vi "RM.searchClientInfoArrayByGUID.vi"(8 "error in (no error)":errorcluster, 10 "ClientGUID":string, 11 "Client Array in":T1[](array[typedef]) {"CD Ref" format="%.0x"}) -> (0 "error out":errorcluster, 1 "found?":bool, 2 "ClientInfo":T1 {"CD Ref" format="%.0x"}, 3 "Client Array out":T1[](array[typedef]) {"CD Ref" format="%.0x"})   [LabVIEW 2016, in "FPGA Resource Manager.lvlib"]
uses:
  FPGA Resource Manager.lvlib
  RM.clientInfo.ctl
  <vilib>/NI Veristand/Custom Device API/Custom Device Item Ref.ctl
  <vilib>/NI Veristand/Custom Device API/Custom Device API.lvlib
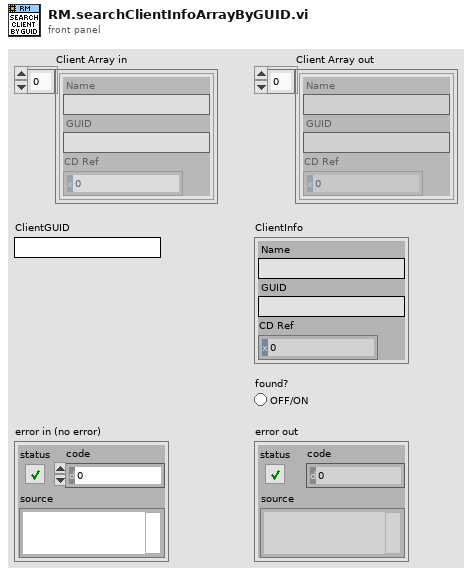
[diagram p1: front panel]
types:
  T1 = typedef "FPGA Resource Manager.lvlib/RM.clientInfo.ctl" = cluster{"Name":string, "GUID":string, "CD Ref":T2}
  T2 = typedef "Custom Device API.lvlib/Custom Device Item Ref.ctl" = u64
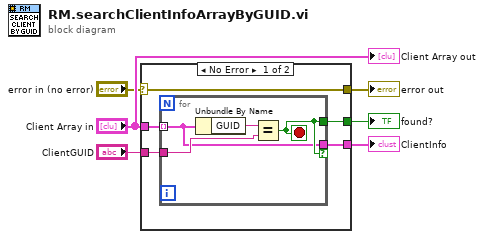
[diagram p0: block diagram]
diagram:
  n1 = case shown="No Error" "error in (no error)" {
    selector: "error in (no error)" -> [w7 w16]
    tunnel: "ClientGUID" -> [w11 _]
    tunnel: "Client Array in" -> [w10 _]
    tunnel: [w9 _] -> w4
    tunnel: [w8 _] -> w3
    tunnel: [w7 w16] -> w1
    frame No Error {
      n2 = for {
        tunnel: w11 -> [w14]
        tunnel: w10 -> [w12] mode=indexing
        tunnel: [w12] -> w9 if=w13
        tunnel: [w13] -> w8
        stop <- w13 stop-if-true
        n3 = Unbundle By Name(w12) -> ("GUID"=w15:string)
        n4 = Equal?(x=w15, y=w14) -> (x = y?=w13:bool)
      }
    }
    frame Error {
    }
  }
  "ClientInfo" <- w4
  "found?" <- w3
  "error out" <- w1
  "Client Array out" <- "Client Array in"
